vi "XML_EEG_readHeader.vi"(8 "error in (no error)":errorcluster, 10 "DOM document in":refnum<k20>, 11 "XML_EEG_Class in":refnum<class "XML_EEG_File.lvclass">) -> (1 "Errors?":bool, 2 "XML Header out":T1, 3 "XML_EEG_Class out":refnum<class "XML_EEG_File.lvclass">)   [LabVIEW 2016, in "XML_EEG_File_Parser.lvlib" / "XML_EEG_File.lvclass"]
uses:
  XML_EEG_File.lvclass
  XML_EEG_Header.ctl
  XML_EEG_File.lvclass/XML_EEG_File.ctl
  <vilib>/xml/NI_XML.lvlib
  XML_EEG_File_Parser.lvlib
panel:
  # "This VI is a part of BCI Design library, http://www.ru-bci.org \nCopyright © 2020, Sotnikov Peter, All rights reserved. License: GNU GPLv3"
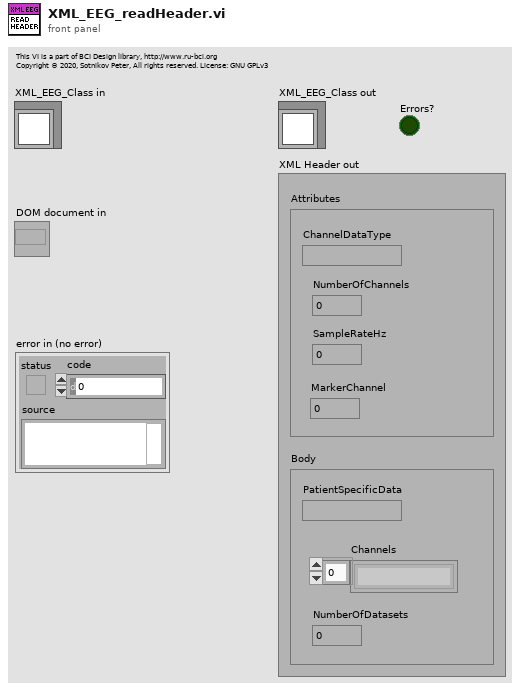
[diagram p1: front panel]
types:
  T1 = typedef "XML_EEG_File_Parser.lvlib/XML_EEG_Header.ctl" = cluster{"Attributes":cluster{"ChannelDataType":string, "NumberOfChannels":i32, "SampleRateHz":dbl, "MarkerChannel":i32}, "Body":cluster{"PatientSpecificData":string, "NumberOfDatasets":i32, "Channels":string[]}}
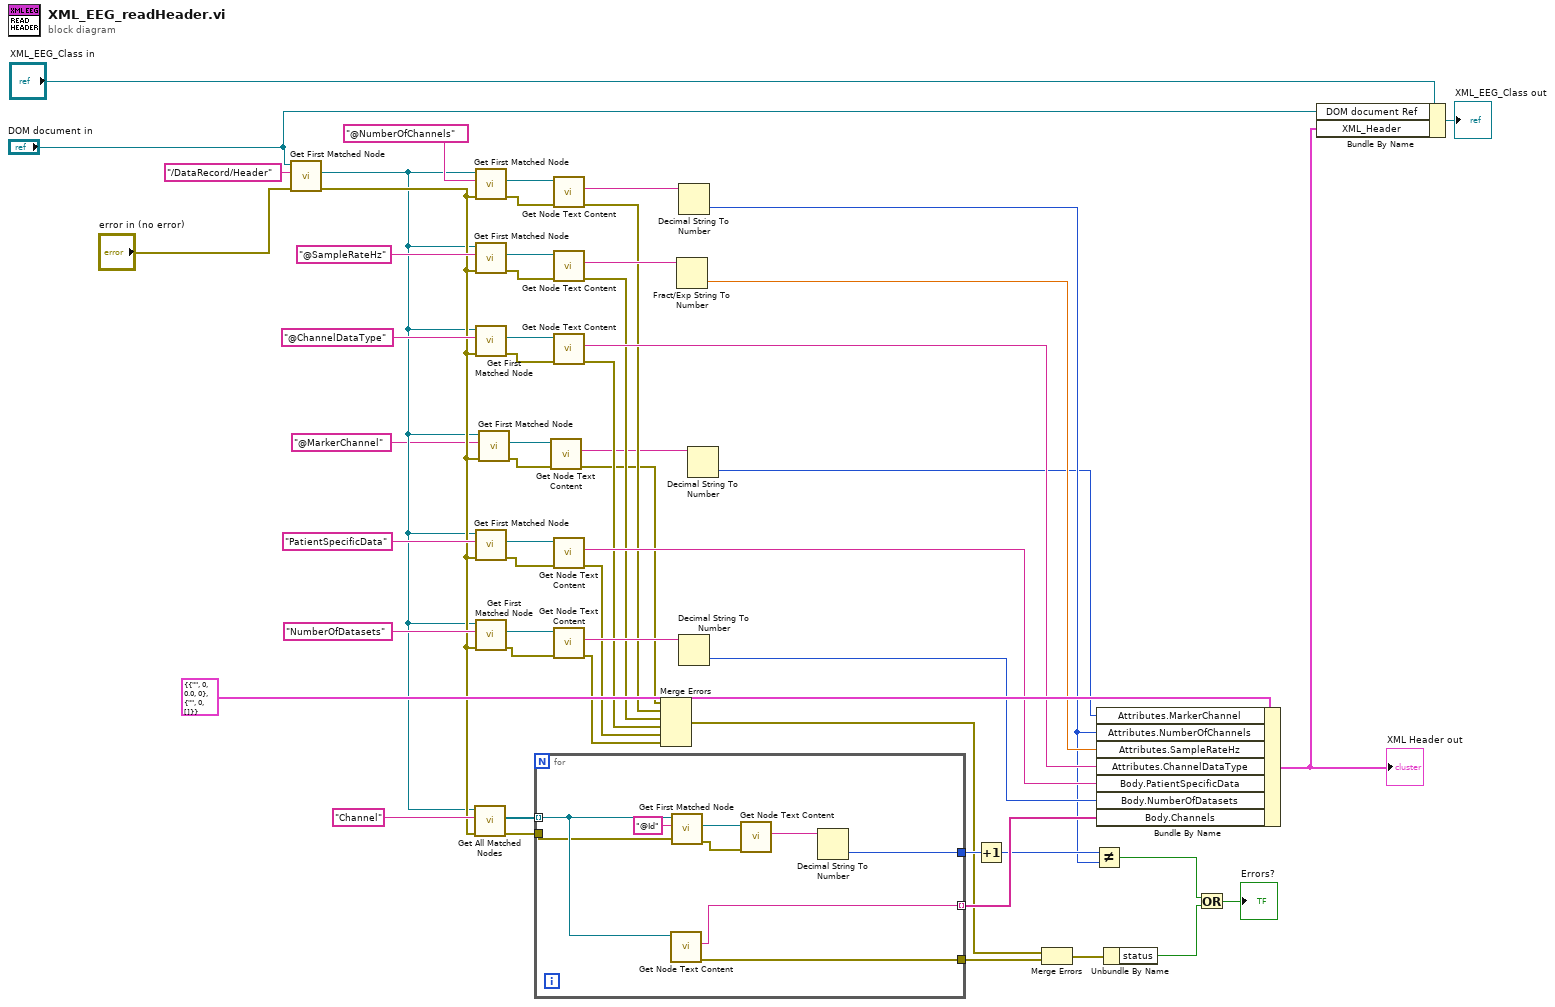
[diagram p0: block diagram]
diagram:
  n1 = call <vilib>:"Get First Matched Node.vi"("error in (no error)"="error in (no error)", "XPath expression"="/DataRecord/Header", "node in"="DOM document in") -> ("error out"=w12:errorcluster, "node result"=w11:refnum<k20>)  [unwired: 6 in, 1 out]
  n2 = call <vilib>:"Get All Matched Nodes.vi"("error in (no error)"=w12, "XPath expression"="Channel", "node in"=w11) -> ("error out"=w29:errorcluster, "node result array"=w28:refnum<k20>[])  [unwired: 6 in, 1 out]
  n3 = call <vilib>:"Get First Matched Node.vi"("error in (no error)"=w12, "XPath expression"="@NumberOfChannels", "node in"=w11) -> ("error out"=w45:errorcluster, "node result"=w52:refnum<k20>)  [unwired: 6 in, 1 out]
  n4 = call <vilib>:"Get First Matched Node.vi"("error in (no error)"=w12, "XPath expression"="@SampleRateHz", "node in"=w11) -> ("error out"=w46:errorcluster, "node result"=w51:refnum<k20>)  [unwired: 6 in, 1 out]
  n5 = call <vilib>:"Get First Matched Node.vi"("error in (no error)"=w12, "XPath expression"="@ChannelDataType", "node in"=w11) -> ("error out"=w47:errorcluster, "node result"=w49:refnum<k20>)  [unwired: 6 in, 1 out]
  n6 = call <vilib>:"Get First Matched Node.vi"("error in (no error)"=w12, "XPath expression"="PatientSpecificData", "node in"=w11) -> ("error out"=w40:errorcluster, "node result"=w41:refnum<k20>)  [unwired: 6 in, 1 out]
  n7 = call <vilib>:"Get First Matched Node.vi"("error in (no error)"=w12, "XPath expression"="NumberOfDatasets", "node in"=w11) -> ("error out"=w39:errorcluster, "node result"=w31:refnum<k20>)  [unwired: 6 in, 1 out]
  n8 = call <vilib>:"Get First Matched Node.vi"("error in (no error)"=w12, "XPath expression"="@MarkerChannel", "node in"=w11) -> ("error out"=w9:errorcluster, "node result"=w8:refnum<k20>)  [unwired: 6 in, 1 out]
  n9 = for {
    tunnel: w29 -> [w61]
    tunnel: w28 -> [w63] mode=indexing
    tunnel: [w56] -> w27 mode=indexing
    tunnel: [w58] -> w26
    tunnel: [w57] -> w18
    n10 = call <vilib>:"Get Node Text Content.vi"("node in"=w63) -> ("error out"=w57:errorcluster, "node text"=w56:string)  [unwired: 8 in, 1 out]
    n11 = call <vilib>:"Get First Matched Node.vi"("error in (no error)"=w61, "XPath expression"="@Id", "node in"=w63) -> ("error out"=w62:errorcluster, "node result"=w60:refnum<k20>)  [unwired: 6 in, 1 out]
    n12 = call <vilib>:"Get Node Text Content.vi"("error in (no error)"=w62, "node in"=w60) -> ("node text"=w59:string)  [unwired: 7 in, 2 out]
    n13 = Decimal String To Number(string=w59) -> (number=w58:i32)  [unwired: 2 in, 1 out]
  }
  n14 = call <vilib>:"Get Node Text Content.vi"("error in (no error)"=w9, "node in"=w8) -> ("error out"=w7:errorcluster, "node text"=w6:string)  [unwired: 7 in, 1 out]
  n15 = call <vilib>:"Get Node Text Content.vi"("error in (no error)"=w45, "node in"=w52) -> ("error out"=w23:errorcluster, "node text"=w44:string)  [unwired: 7 in, 1 out]
  n16 = call <vilib>:"Get Node Text Content.vi"("error in (no error)"=w46, "node in"=w51) -> ("error out"=w22:errorcluster, "node text"=w43:string)  [unwired: 7 in, 1 out]
  n17 = call <vilib>:"Get Node Text Content.vi"("error in (no error)"=w47, "node in"=w49) -> ("error out"=w21:errorcluster, "node text"=w34:string)  [unwired: 7 in, 1 out]
  n18 = call <vilib>:"Get Node Text Content.vi"("error in (no error)"=w40, "node in"=w41) -> ("error out"=w20:errorcluster, "node text"=w33:string)  [unwired: 7 in, 1 out]
  n19 = call <vilib>:"Get Node Text Content.vi"("error in (no error)"=w39, "node in"=w31) -> ("error out"=w19:errorcluster, "node text"=w37:string)  [unwired: 7 in, 1 out]
  n20 = Merge Errors(w7, w23, w22, w21, w20, w19) -> (w17:errorcluster)
  n21 = Fract/Exp String To Number(string=w43) -> (number=w35:dbl)  [unwired: 3 in, 1 out]
  n22 = Decimal String To Number(string=w44) -> (number=w24:i32)  [unwired: 2 in, 1 out]
  n23 = Decimal String To Number(string=w37) -> (number=w32:i32)  [unwired: 2 in, 1 out]
  n24 = Decimal String To Number(string=w6) -> (number=w5:i32)  [unwired: 2 in, 1 out]
  n25 = Increment(x=w26) -> (x+1=w25:i32)
  n26 = Merge Errors(w17, w18) -> (w16:errorcluster)
  n27 = Not Equal?(x=w25, y=w24) -> (x != y?=w15:bool)
  n28 = Bundle By Name(cluster=T1 {"Attributes"={"ChannelDataType"="", "NumberOfChannels"=0, "SampleRateHz"=0.0, "MarkerChannel"=0}, "Body"={"PatientSpecificData"="", "NumberOfDatasets"=0, "Channels"=[]}} ("XML_Header"), "Attributes.MarkerChannel"=w5, "Attributes.NumberOfChannels"=w24, "Attributes.SampleRateHz"=w35, "Attributes.ChannelDataType"=w34, "Body.PatientSpecificData"=w33, "Body.NumberOfDatasets"=w32, "Body.Channels"=w27) -> (w2:T1)
  "XML Header out" <- w2
  n29 = Unbundle By Name(w16) -> ("status"=w14:bool)
  n30 = Or(x=w15, y=w14) -> (x .or. y?=→"Errors?":bool)
  n31 = Bundle By Name(cluster="XML_EEG_Class in", "DOM document Ref"="DOM document in", "XML_Header"=w2) -> (→"XML_EEG_Class out":refnum<class "XML_EEG_File.lvclass">)
